vi "Test (API Reflection).vi"() -> ()   [LabVIEW 2015]
uses:
  SLSC Remote Interface Class/Initialize (Remote Device).vi
  SLSC Interface Class/Open Command/Open Device Command.vi
  SLSC Interface Class/Open Property/Open Device Property.vi
  SLSC Remote Interface Class/SLSC Remote.lvclass
  SLSC Interface Class/SLSC Interface.lvclass
panel:
  out "command error out":errorcluster
  out "property error out":errorcluster
  out "Cmd.Doc":string
  out "Cmd.Descr":string
  out "Prop.Enum.Name":string
  out "Prop.Enum.ValueNames":string[](array[string])
  out "Prop.Enum.Values":i32[](array[numeric])
  out "Prop.IsEnum":bool
  out "Prop.Descr":string
  out "session error out":errorcluster
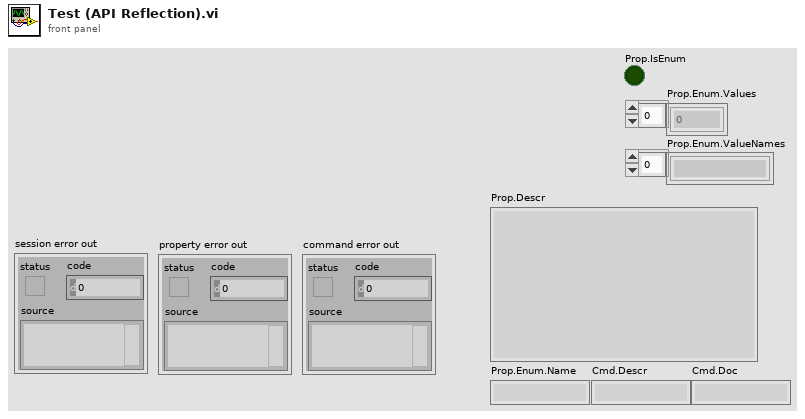
[diagram p1: front panel]
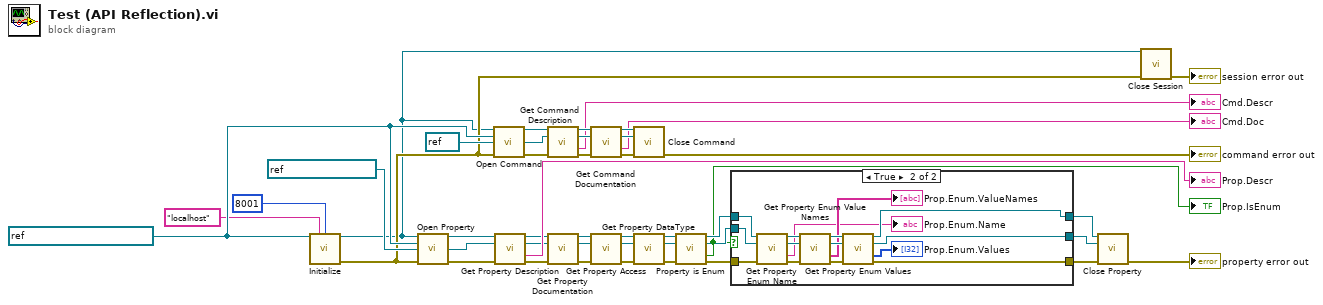
[diagram p0: block diagram]
diagram:
  w10 = refnum<k21> "SLSC-12001-030EE1BD" ("devices")
  n1 = call-poly "Initialize.vi"("devices"=w10, "Hostname/IP"="localhost", "Port"=u16 8001) -> ("SLSC Remote out"=w1:refnum<class "SLSC Remote.lvclass">, "error out"=w6:errorcluster)  [unwired: 11 in]
  n2 = call-poly "Open Property.vi"("SLSC Interface in"=w1, "device"=w10, "property in"=refnum<k21> "PowerOnHours", "error in (no error)"=w6) -> ("SLSC Interface out"=w42:refnum<class "SLSC Remote.lvclass">, "property out"=w40:refnum<k21>, "error out"=w41:errorcluster)  [unwired: 9 in]
  n3 = call-poly "Open Command.vi"("SLSC Interface in"=w1, "device"=w10, "command in"=refnum<k21> refnum, "error in (no error)"=w6) -> ("SLSC Interface out"=w19:refnum<class "SLSC Remote.lvclass">, "command out"=w16:refnum<k21>, "error out"=w11:errorcluster)  [unwired: 9 in]
  n4 = call-dynamic "Get Property Description.vi"("SLSC Remote in"=w42, "property"=w40, "error in (no error)"=w41) -> ("SLSC Remote out"=w30:refnum<class "SLSC Remote.lvclass">, "property out"=w21:refnum<k21>, "Prop.Descr"=→"Prop.Descr":string, "error out"=w29:errorcluster)  [unwired: 9 in]
  n5 = call-dynamic "Get Command Description.vi"("SLSC Remote in"=w19, "command in"=w16, "error in (no error)"=w11) -> ("SLSC Remote out"=w18:refnum<class "SLSC Remote.lvclass">, "command out"=w15:refnum<k21>, "Cmd.Descr"=→"Cmd.Descr":string, "error out"=w12:errorcluster)  [unwired: 9 in]
  n6 = call-dynamic "Get Property Documentation.vi"("SLSC Remote in"=w30, "property"=w21, "error in (no error)"=w29) -> ("SLSC Remote out"=w38:refnum<class "SLSC Remote.lvclass">, "property out"=w28:refnum<k21>, "error out"=w37:errorcluster)  [unwired: 9 in, 1 out]
  n7 = call-dynamic "Get Command Documentation.vi"("SLSC Remote in"=w18, "command"=w15, "error in (no error)"=w12) -> ("SLSC Remote out"=w17:refnum<class "SLSC Remote.lvclass">, "command out"=w14:refnum<k21>, "Cmd.Doc"=→"Cmd.Doc":string, "error out"=w13:errorcluster)  [unwired: 9 in]
  n8 = call-dynamic "Get Property Access.vi"("SLSC Remote in"=w38, "property"=w28, "error in (no error)"=w37) -> ("SLSC Remote out"=w36:refnum<class "SLSC Remote.lvclass">, "property out"=w27:refnum<k21>, "error out"=w35:errorcluster)  [unwired: 9 in, 1 out]
  n9 = call-dynamic "Close Command.vi"("SLSC Remote in"=w17, "command"=w14, "error in (no error)"=w13) -> ("error out"=→"command error out":errorcluster)  [unwired: 11 in, 1 out]
  n10 = call-dynamic "Get Property DataType.vi"("SLSC Remote in"=w36, "property"=w27, "error in (no error)"=w35) -> ("SLSC Remote out"=w34:refnum<class "SLSC Remote.lvclass">, "property out"=w22:refnum<k21>, "error out"=w33:errorcluster)  [unwired: 9 in, 1 out]
  n11 = call-dynamic "Property is Enum.vi"("SLSC Remote in"=w34, "property"=w22, "error in (no error)"=w33) -> ("SLSC Remote out"=w32:refnum<class "SLSC Remote.lvclass">, "property out"=w23:refnum<k21>, "Prop.IsEnum"=w20:bool, "error out"=w31:errorcluster)  [unwired: 9 in]
  "Prop.IsEnum" <- w20
  n12 = case shown="True" w20 {
    tunnel: w32 -> [w47 w62]
    tunnel: w31 -> [w45 w61]
    tunnel: [w47 w56] -> w26
    tunnel: [w45 w55] -> w25
    tunnel: [w46 w54] -> w24
    tunnel: w23 -> [w46 w51]
    frame False {
    }
    frame True {
      n13 = call-dynamic "Get Property Enum Name.vi"("SLSC Remote in"=w62, "property"=w51, "error in (no error)"=w61) -> ("SLSC Remote out"=w60:refnum<class "SLSC Remote.lvclass">, "property out"=w52:refnum<k21>, "Prop.Enum.Name"=→"Prop.Enum.Name":string, "error out"=w59:errorcluster)  [unwired: 9 in]
      n14 = call-dynamic "Get Property Enum Value Names.vi"("SLSC Remote in"=w60, "property"=w52, "error in (no error)"=w59) -> ("SLSC Remote out"=w58:refnum<class "SLSC Remote.lvclass">, "property out"=w53:refnum<k21>, "Prop.Enum.ValueNames"=→"Prop.Enum.ValueNames":string[], "error out"=w57:errorcluster)  [unwired: 9 in]
      n15 = call-dynamic "Get Property Enum Values.vi"("SLSC Remote in"=w58, "property"=w53, "error in (no error)"=w57) -> ("SLSC Remote out"=w56:refnum<class "SLSC Remote.lvclass">, "property out"=w54:refnum<k21>, "Prop.Enum.Values"=→"Prop.Enum.Values":i32[], "error out"=w55:errorcluster)  [unwired: 9 in]
    }
  }
  n16 = call-dynamic "Close Property.vi"("SLSC Remote in"=w26, "property"=w24, "error in (no error)"=w25) -> ("error out"=→"property error out":errorcluster)  [unwired: 11 in, 1 out]
  n17 = call-dynamic "Close Session.vi"("SLSC Remote in"=w1, "error in (no error)"=w6) -> ("error out"=→"session error out":errorcluster)  [unwired: 13 in]
